vi "Queue Access FGV.vi"(6 "FGV State Command":T1, 8 "error in (no error)":errorcluster) -> (0 "error out":errorcluster, 3 "queue out":refnum<queue>)   [LabVIEW 2021]
uses:
  Typedefs/Q FGV State Command.ctl
  Typedefs/Q Message Data.ctl
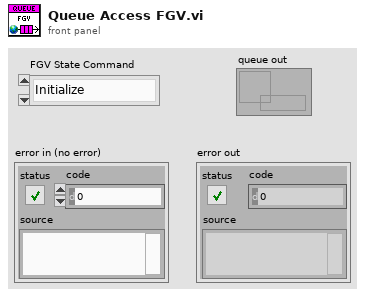
[diagram p1: front panel]
types:
  T1 = typedef "Q FGV State Command.ctl" = enum16{"Initialize", "Get", "Release"}
  T2 = typedef "Q Message Data.ctl" = cluster{"State Command":string, "Data":variant}
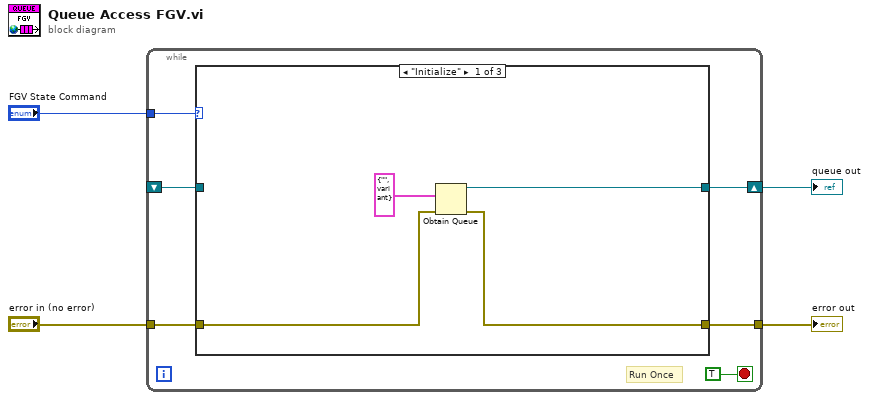
[diagram p0: block diagram]
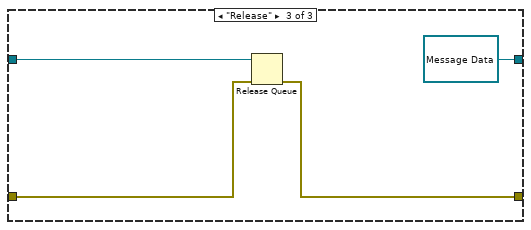
[diagram p3: hidden frame]
diagram:
  n1 = while {
    tunnel: "FGV State Command" -> [w9]
    tunnel: "error in (no error)" -> [w8]
    tunnel: [w7] -> w1
    shift-right: [w6] -> w3
    shift-left: _ -> [w5]
    stop <- TRUE stop-if-true
    # "Run Once"
    n2 = case shown="\"Initialize\"" w9 {
      tunnel: w8 -> [w14 w15 w19]
      tunnel: [w13 w15 w18] -> w7
      tunnel: [w12 w16 refnum<queue> refnum ("queue out")] -> w6
      tunnel: w5 -> [_ w16 w20]
      frame "Initialize" {
        n3 = Obtain Queue(element data type=T2 {"State Command"="", "Data"=variant} ("Message Data"), error in (no error)=w14) -> (queue out=w12:refnum<queue>, error out=w13:errorcluster)  [unwired: 3 in, 1 out]
      }
      frame "Get", Default {
      }
      frame "Release" {
        n4 = Release Queue(queue=w20, error in (no error)=w19) -> (error out=w18:errorcluster)  [unwired: 1 in, 2 out]
      }
    }
  }
  "queue out" <- w3
  "error out" <- w1
